vi "Test_monitorCommand_setArrays.vi"(8 "error in (no error)":errorcluster, 11 "command_setArrays_Ctl":T1={"boolean0[5]"=[FALSE, FALSE, FALSE, FALSE, FALSE], "byte0[5]"=[0, 0, 0, 0, 0], "char0"="", "short0[5]"=[0, 0, 0, 0, 0], "int0[5]"=[0, 0, 0, 0, 0], "long0[5]"=[0, 0, 0, 0, 0], "longLong0[5]"=[0, 0, 0, 0, 0], "octet0[5]"=[0, 0, 0, 0, 0], "unsignedShort0[5]"=[0, 0, 0, 0, 0], "unsignedInt0[5]"=[0, 0, 0, 0, 0], "unsignedLong0[5]"=[0, 0, 0, 0, 0], "float0[5]"=[0.0, 0.0, 0.0, 0.0, 0.0], "double0[5]"=[0.0, 0.0, 0.0, 0.0, 0.0]}) -> (0 "error out":errorcluster, 2 "function return":i32, 3 "command_setArrays_Ctl out":T1)   [LabVIEW 2016, in "SALLV_Test.lvlib"]
doc: "int Test_shm_monitorCommand_setArraysLV(Test_command_setArraysLV *command_setArrays_Ctl );"
uses:
  SALLV_Test.lvlib
  DataTypes/command_setArrays.ctl
  SALLV_Test.so
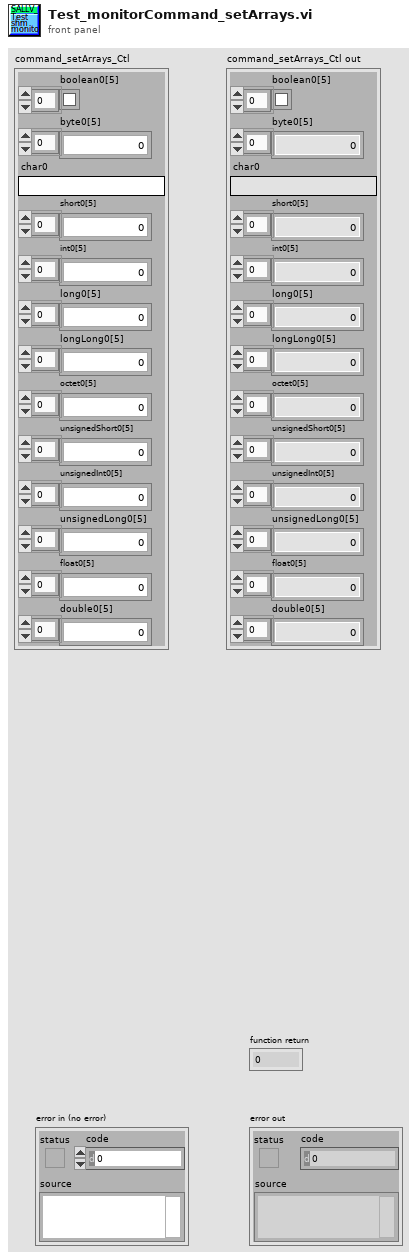
[diagram p1: front panel]
types:
  T1 = typedef "SALLV_Test.lvlib/command_setArrays.ctl" = cluster{"boolean0[5]":bool[], "byte0[5]":u8[], "char0":string, "short0[5]":i16[], "int0[5]":i32[], "long0[5]":i32[], "longLong0[5]":i64[], "octet0[5]":u8[], "unsignedShort0[5]":u16[], "unsignedInt0[5]":u32[], "unsignedLong0[5]":u32[], "float0[5]":sgl[], "double0[5]":dbl[]}
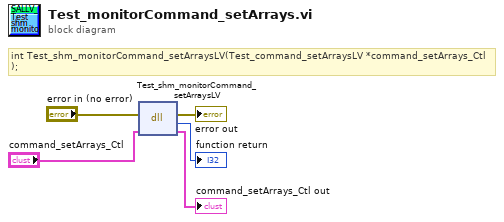
[diagram p0: block diagram]
diagram:
  # "int Test_shm_monitorCommand_setArraysLV(Test_command_setArraysLV *command_setArrays_Ctl );"
  n1 = dll-call lib="home/ccontaxis/Code/SALLV_Test/SALLV_Test.*" fn="Test_shm_monitorCommand_setArraysLV"(error in="error in (no error)", "command_setArrays_Ctl"="command_setArrays_Ctl") -> (error out=→"error out":errorcluster, →"function return":i32, "command_setArrays_Ctl"=→"command_setArrays_Ctl out":T1)  [unwired: 2 in, 1 out]
